vi "Calc XYZbar_j.vi"(8 "theta_j":dbl, 9 "j":i32, 11 "Analytical Serial Arm Class in":refnum<class "NI_Robotics_Analytical Serial Arm Class.lvclass">) -> (2 "XYZbar_j":dbl[](array[numeric]), 3 "Analytical Serial Arm Class out":refnum<class "NI_Robotics_Analytical Serial Arm Class.lvclass">)   [LabVIEW 2017, in "NI_Robotics_Analytical Serial Arm Class.lvclass"]
uses:
  <vilib>/robotics/Kinematics/Analytical/Generic/NI_Robotics_Analytical Serial Arm Class.lvclass
  c:/Program Files (x86)/National Instruments/LabVIEW 2017/vi.lib/robotics/Kinematics/Robot/NI_Robotics_Serial Robot Arm.lvclass
  <vilib>/robotics/Kinematics/Link/NI_Robotics_Link.lvclass/NI_Robotics_Link.ctl
  <vilib>/robotics/Kinematics/Link/Get Kinematic Parameters.vi
  <vilib>/robotics/Kinematics/Analytical/Generic/Accessors/Read alpha_n0.vi
  <vilib>/robotics/Kinematics/Robot/Get Links.vi
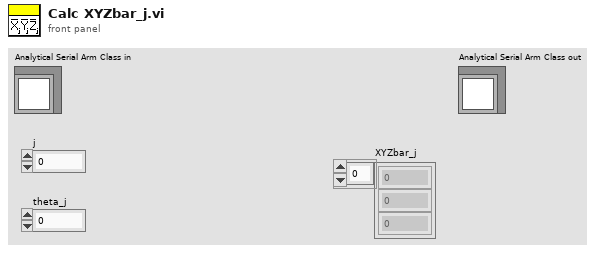
[diagram p1: front panel]
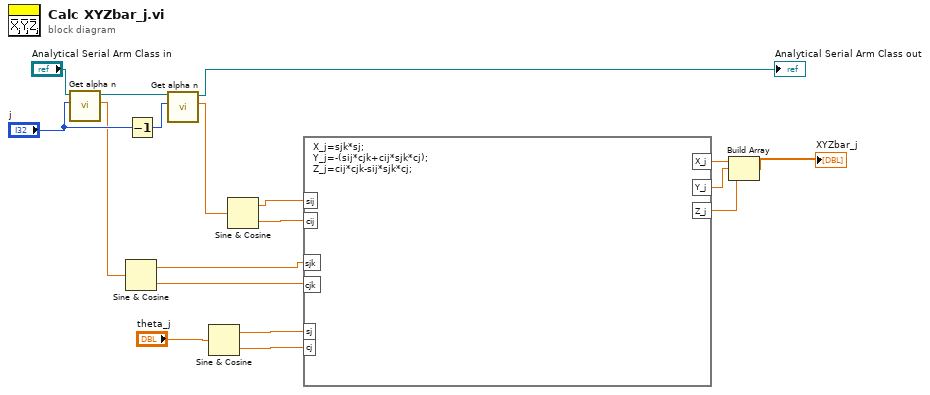
[diagram p0: block diagram]
diagram:
  n1 = call <vilib>:"Get alpha n.vi"("n"="j", "Analytical Serial Arm Class in"="Analytical Serial Arm Class in") -> ("alpha n"=w6:dbl, "Analytical Serial Arm Class out"=w11:refnum<class "NI_Robotics_Analytical Serial Arm Class.lvclass">)  [unwired: 8 in]
  n2 = Sine & Cosine(0:w6) -> (1:w18:dbl, 2:w17:dbl)
  n3 = Decrement(x="j") -> (x-1=w7:i32)
  n4 = call <vilib>:"Get alpha n.vi"("n"=w7, "Analytical Serial Arm Class in"=w11) -> ("alpha n"=w5:dbl, "Analytical Serial Arm Class out"=→"Analytical Serial Arm Class out":refnum<class "NI_Robotics_Analytical Serial Arm Class.lvclass">)  [unwired: 8 in]
  n5 = Sine & Cosine(0:"theta_j") -> (1:w13:dbl, 2:w12:dbl)
  n6 = Sine & Cosine(0:w5) -> (1:w15:dbl, 2:w16:dbl)
  n7 = formula code="X_j=sjk*sj;\nY_j=-(sij*cjk+cij*sjk*cj);\nZ_j=cij*cjk-sij*sjk*cj;"("sij"=w15, "cij"=w16, "sjk"=w18, "cjk"=w17, "sj"=w13, "cj"=w12) -> ("X_j"=w4:dbl, "Y_j"=w3:dbl, "Z_j"=w2:dbl)
  n8 = Build Array(w4, w3, w2) -> (→"XYZbar_j":dbl[])
